vi "Configure IScan Trigger (Runt).vi"(0 "VISA resource name":refnum<visa-resource-name>, 1 "Lower Level Limit (0 V)":dbl, 5 "Channel (1: Channel1)":i32(ring)=1 items=["Channel1"=1, "Channel2"=2, "Channel3"=3, "Channel4"=4], 7 "Hysteresis Value (0 V)":dbl, 11 "error in (no error)":errorcluster, 12 "Upper Level Limit (0.01 V)":dbl=0.01) -> (4 "VISA resource name out":refnum<visa-resource-name>="DSO90604A", 15 "error out":errorcluster)   [LabVIEW 2020, in "Agilent 90000 Series.lvlib"]
doc: "Configures InfiniiScan trigger under runt trigger mode."
uses:
  Agilent 90000 Series.lvlib
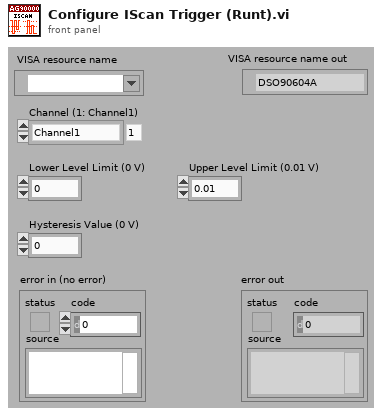
[diagram p1: front panel]
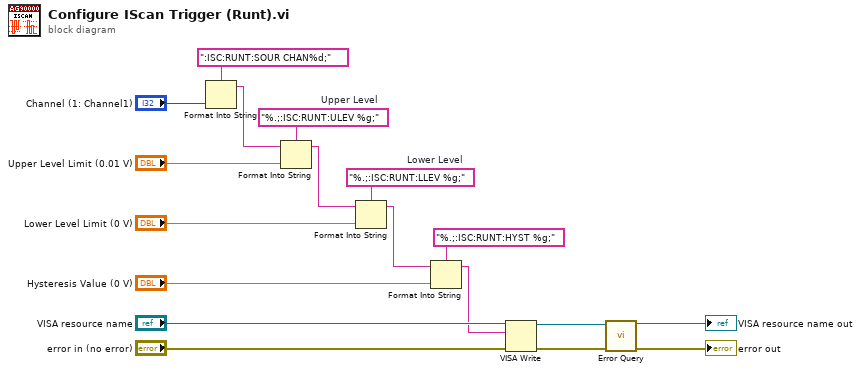
[diagram p0: block diagram]
diagram:
  w13 = "%.;:ISC:RUNT:LLEV %g;"  # Lower Level
  w15 = "%.;:ISC:RUNT:ULEV %g;"  # Upper Level
  n1 = Format Into String(format string=":ISC:RUNT:SOUR CHAN%d;", "Channel (1: Channel1)") -> (resulting string=w16:string)  [unwired: 2 in, 1 out]
  n2 = Format Into String(format string=w15, initial string=w16, "Upper Level Limit (0.01 V)") -> (resulting string=w3:string)  [unwired: 1 in, 1 out]
  n3 = Format Into String(format string=w13, initial string=w3, "Lower Level Limit (0 V)") -> (resulting string=w2:string)  [unwired: 1 in, 1 out]
  n4 = Format Into String(format string="%.;:ISC:RUNT:HYST %g;", initial string=w2, "Hysteresis Value (0 V)") -> (resulting string=w1:string)  [unwired: 1 in, 1 out]
  n5 = VISA Write(VISA resource name="VISA resource name", write buffer=w1, error in (no error)="error in (no error)") -> (VISA resource name out=w7:refnum<visa-resource-name>, error out=w6:errorcluster)  [unwired: 1 out]
  n6 = call "Error Query.vi"("error in (no error)"=w6, "VISA resource name"=w7) -> ("error out"=→"error out":errorcluster, "VISA resource name out"=→"VISA resource name out":refnum<visa-resource-name>)  [unwired: 8 out]
